vi "MR16 Test Stand - main.vi"() -> ()   [LabVIEW 2013]
doc: "Use this template to build a standard state machine design pattern. Each state executes code and determines which state to transition to. Contrast this design pattern with the User Interface Event Handler pattern, in which code executes in response to user actions. Contrast this design pattern also with the Queued Message Handler pattern, in which each message handling code can queue zero or more new messages."
uses:
  Controls/Test Case.ctl
  Controls/arranged waveforms.ctl
  Controls/waveform display.ctl
  Controls/Data Cluster.ctl
  Controls/Power Values.ctl
  <vilib>/addons/Electrical Power/Basic/Measurement/subVIs/basic_Power Value.ctl
  Controls/Stabilization.ctl
  Controls/StateMachineStates 1.ctl
  <vilib>/addons/Electrical Power/Basic/NI_EP_Basic.lvlib
panel:
  out "Test Case 2":T1
  out "Data Cluster":T2
  out "Waveforms":T6
  out "error out":errorcluster
  in  "Send Notifier Emails?":bool
  out "Status":string
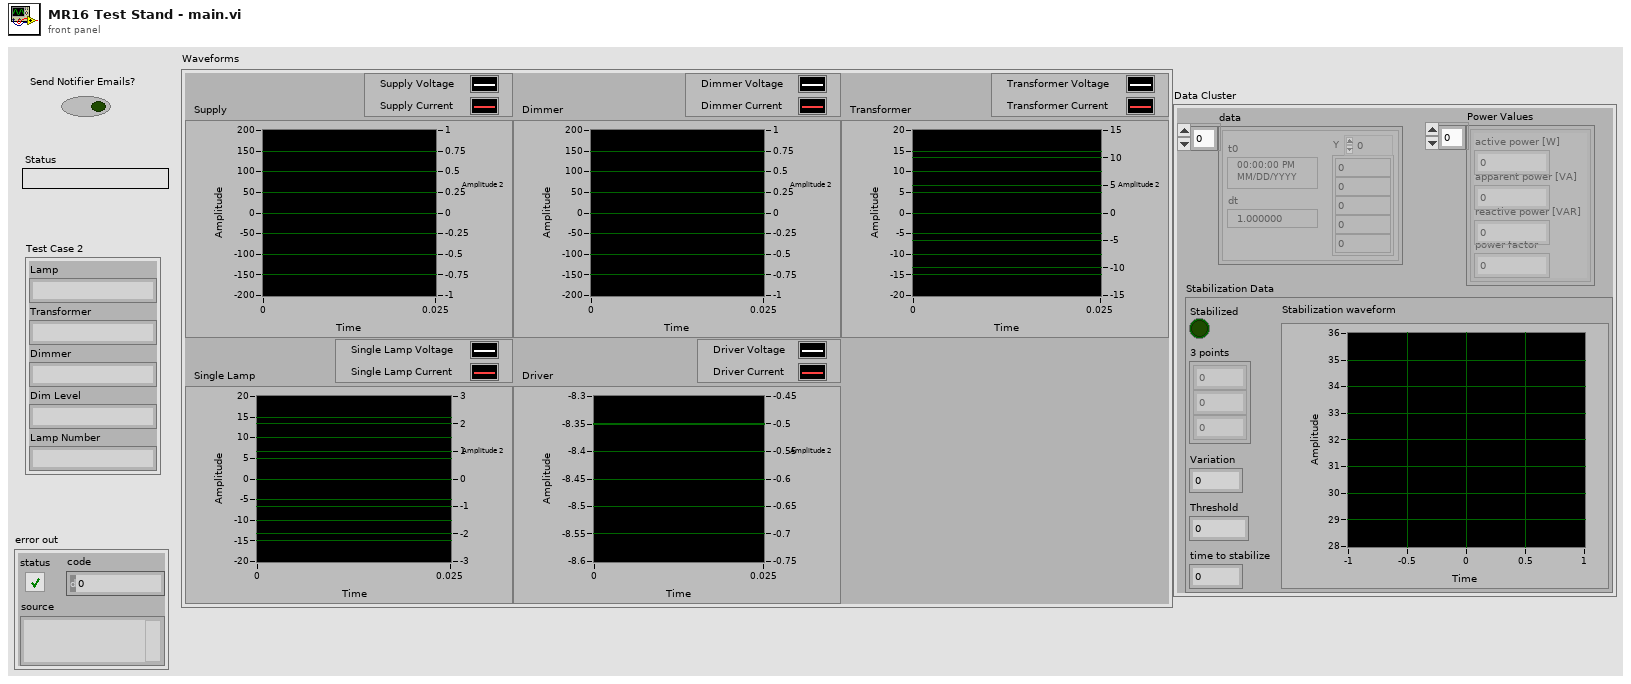
[diagram p1: front panel]
types:
  T1 = typedef "Test Case.ctl" = cluster{"Lamp":string, "Transformer":string, "Dimmer":string, "Dim Level":string, "Lamp Number":string}
  T2 = typedef "Data Cluster.ctl" = cluster{"data":waveform(dbl)[], "Power Values":T3, "Stabilization Data":T5}
  T3 = typedef "Power Values.ctl" = T4[]
  T4 = typedef "NI_EP_Basic.lvlib/basic_Power Value.ctl" = cluster{"active power [W]":dbl, "apparent power [VA]":dbl, "reactive power [VAR]":dbl, "power factor":dbl}
  T5 = typedef "Stabilization.ctl" = cluster{"Stabilization waveform":waveform(dbl), "Variation":dbl, "Stabilized":bool, "Threshold":dbl, "time to stabilize":dbl, "3 points":dbl[]}
  T6 = typedef "arranged waveforms.ctl" = cluster{"Supply":T7, "Dimmer":T7, "Transformer":T7, "Single Lamp":T7, "Driver":T7}
  T7 = typedef "waveform display.ctl" = waveform(dbl)[]
  T8 = typedef "StateMachineStates 1.ctl" = enum16{"Initialize", "Idle", "determine next test case", "Set Dimmer", "Stabilize and Measure", "notify operator", "Stop"}
  T9 = typedef "data.ctl" = cluster{"index":i32, "all rows":string[][]}
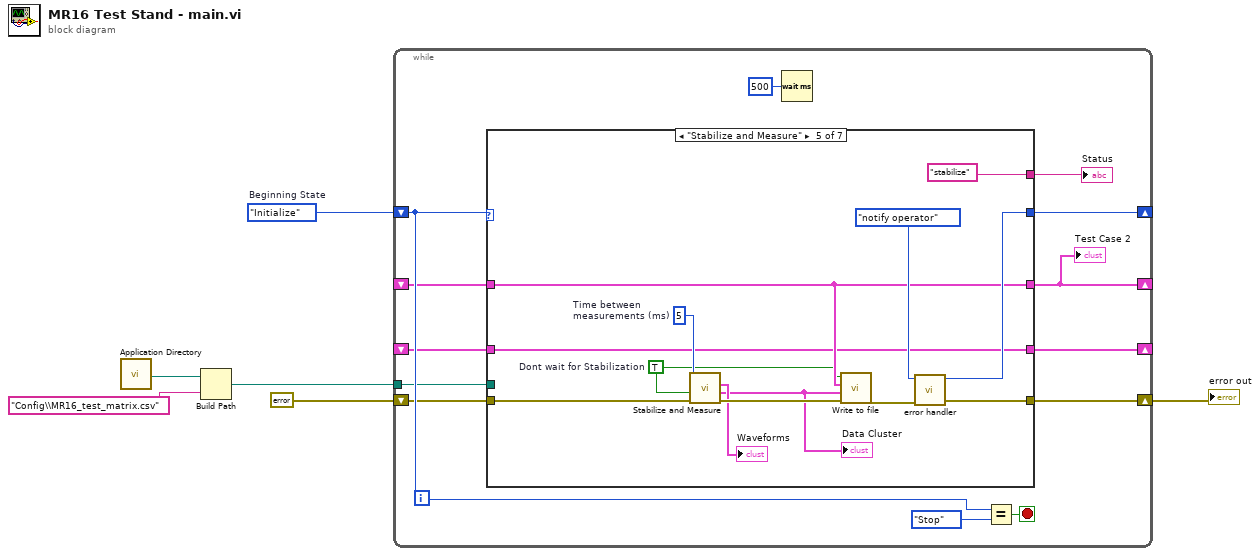
[diagram p0: block diagram]
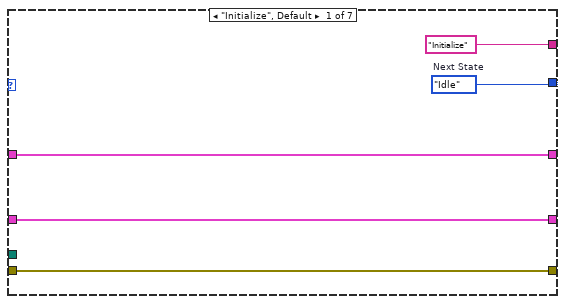
[diagram p2: hidden frame]
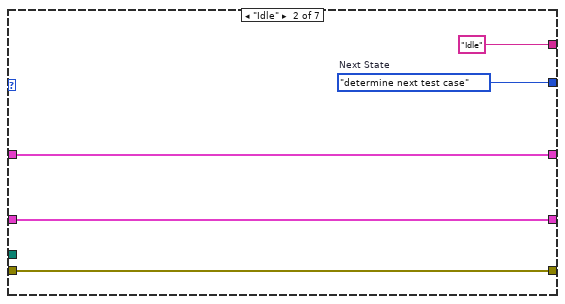
[diagram p3: hidden frame]
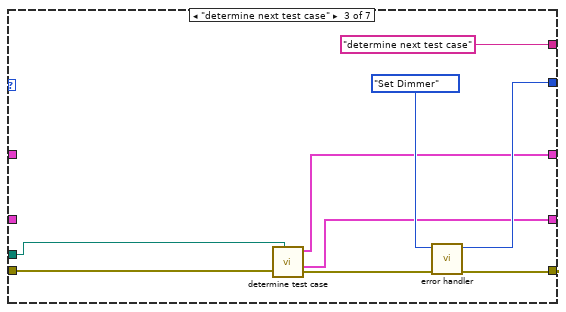
[diagram p4: hidden frame]
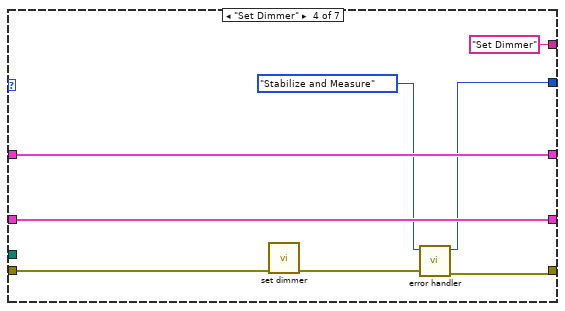
[diagram p5: hidden frame]
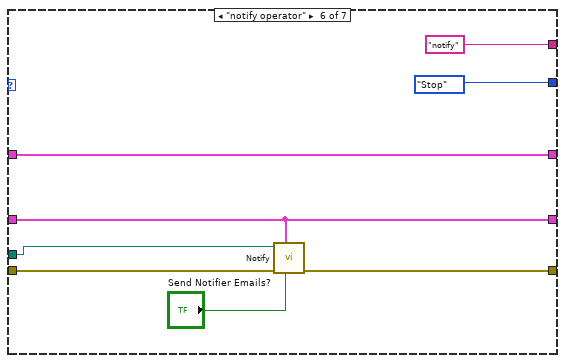
[diagram p6: hidden frame]
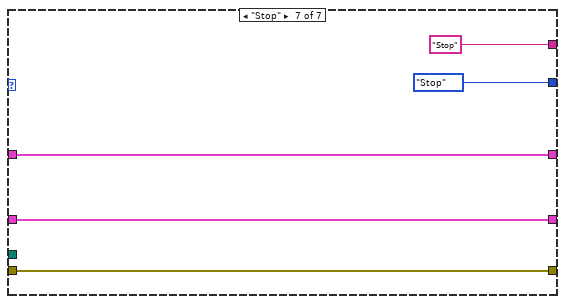
[diagram p7: hidden frame]
diagram:
  w6 = StateMachineStates_1."Initialize"  # Beginning State
  n1 = call <vilib>:"Application Directory.vi"() -> ("Application Directory"=w4:path)
  n2 = Build Path(base path=w4, name or relative path="Config\\MR16_test_matrix.csv") -> (appended path=w3:path)
  n3 = while {
    shift-right: [w16] -> _
    shift-left: w6 -> [w17]
    tunnel: w3 -> [w10]
    shift-right: [w12] -> w1
    shift-left: errorcluster {"status"=FALSE, "code"=0, "source"=""} ("error constant") -> [w13]
    shift-right: [w7] -> _
    shift-left: _ -> [w11]
    shift-right: [w8] -> _
    shift-left: _ -> [w9]
    stop <- w19 stop-if-true
    n4 = case shown="\"Stabilize and Measure\"" w17 {
      tunnel: [w24 w27 w35 w39 w54 StateMachineStates_1."Stop" ("Next State") StateMachineStates_1."Stop" ("Next State")] -> w16
      tunnel: ["Initialize" "Idle" "determine next test case" "Set Dimmer" "stabilize" "notify" "Stop"] -> w14
      tunnel: w13 -> [w22 w28 w37 w45 w58 w64 w70]
      tunnel: [w22 w28 w34 w41 w56 w63 w70] -> w12
      tunnel: [w21 w26 w33 w44 w51 w62 w69] -> w8
      tunnel: w11 -> [w20 w25 _ w43 w50 w61 w68]
      tunnel: [w20 w25 w31 w43 w50 w61 w68] -> w7
      tunnel: w10 -> [_ _ w32 _ _ w65 _]
      tunnel: w9 -> [w21 w26 _ w44 w51 w62 w69]
      frame "Initialize", Default {
        w24 = StateMachineStates_1."Idle"  # Next State
      }
      frame "Idle" {
        w27 = StateMachineStates_1."determine next test case"  # Next State
      }
      frame "determine next test case" {
        n5 = call "determine test case.vi"("error in"=w37, "file path (dialog if empty)"=w32) -> ("error out"=w30:errorcluster, "Test Matrix Data"=w31:T9, "Test Case Cluster"=w33:T1)  [unwired: 7 in]
        n6 = call "error handler.vi"("error in (no error)"=w30, "Next State in"=StateMachineStates_1."Set Dimmer" ("Next State")) -> ("error out"=w34:errorcluster, "Next State out"=w35:T8)  [unwired: 8 in]
      }
      frame "Set Dimmer" {
        n7 = call "set dimmer.vi"("error in"=w45) -> ("error out"=w42:errorcluster)  [unwired: 9 in, 1 out]
        n8 = call "error handler.vi"("error in (no error)"=w42, "Next State in"=StateMachineStates_1."Stabilize and Measure" ("Next State")) -> ("error out"=w41:errorcluster, "Next State out"=w39:T8)  [unwired: 8 in]
      }
      frame "Stabilize and Measure" {
        w49 = TRUE  # Dont wait for Stabilization
        w57 = u32 5  # Time between measurements (ms)
        n9 = call "Stabilize and Measure.vi"("error in"=w58, "Dont wait for Stabilization"=w49, "Time between\nmeasurements (s)"=w57) -> ("error out"=w53:errorcluster, "Data Cluster"=w47:T2, "Waveforms"=→"Waveforms":T6)  [unwired: 6 in]
        "Data Cluster" <- w47
        n10 = call "Write to file.vi"("error in (no error)"=w53, "Data Cluster"=w47, "Test Case"=w51, "Don't wait for stabilizatoin"=w49) -> ("error out"=w52:errorcluster)  [unwired: 7 in]
        n11 = call "error handler.vi"("error in (no error)"=w52, "Next State in"=StateMachineStates_1."notify operator" ("Next State")) -> ("error out"=w56:errorcluster, "Next State out"=w54:T8)  [unwired: 8 in]
      }
      frame "notify operator" {
        n12 = call "Notify.vi"("Send Notifier Emails?"="Send Notifier Emails?", "Test Matrix"=w61, "error in (no error)"=w64, "appended path"=w65) -> ("error out"=w63:errorcluster)  [unwired: 6 in]
      }
      frame "Stop" {
      }
    }
    "Status" <- w14
    "Test Case 2" <- w8
    n13 = Wait (ms)(milliseconds to wait=u32 500) -> ()  [unwired: 1 out]
    n14 = Equal?(x=w17, y=StateMachineStates_1."Stop" ("States")) -> (x = y?=w19:bool)
  }
  "error out" <- w1
